vi "Measure List Report.vi"(8 "error in":errorcluster, 10 "List Number":i32(ring) items=["List 1", "List 2", "List 3", "List 4"], 11 "Instrument Handle In":i32) -> (0 "error out":errorcluster, 2 "Result":dbl[](array[numeric]), 3 "Instrument Handle Out":i32)   [LabVIEW 8.6, in "ZTScopeM.lvlib"]
doc: "Query the measurement results in a measurement list."
uses:
  ZTScopeM.lvlib
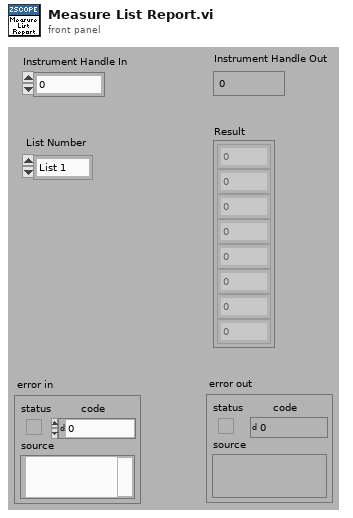
[diagram p1: front panel]
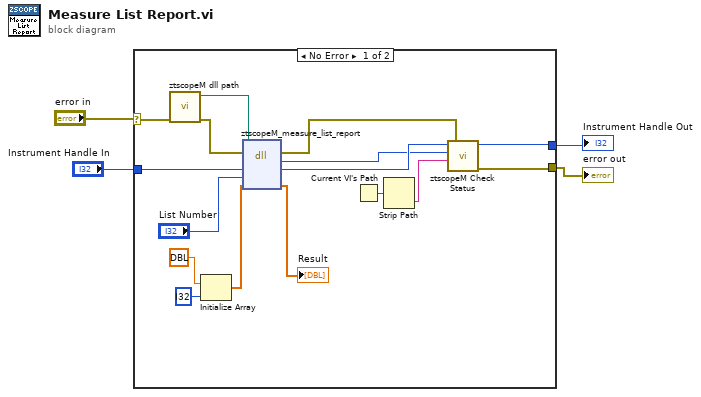
[diagram p0: block diagram]
diagram:
  n1 = case shown="No Error" "error in" {
    selector: "error in" -> [w8 w22]
    tunnel: [w13 w22] -> w1
    tunnel: [w12 w21] -> w4
    tunnel: "Instrument Handle In" -> [w19 w21]
    frame #0 {
      n2 = call "ztscopeM dll path.vi"("error in (no error)"=w8) -> ("error out"=w6:errorcluster, "<instrument>.dll path"=w7:path)  [unwired: 9 in]
      n3 = Initialize Array(dbl ?, i32 ? ("dimension size")) -> (w9:dbl[])
      n4 = dll-call lib="C:/Program Files (x86)/National Instruments/LabVIEW 2013/instr.lib/ztscopem/ztscopeM.dll" fn="ztscopeM_measure_list_report"(path in=w7, error in=w6, "instrumentHandle"=w19, "listNumber"="List Number", "result"=w9) -> (error out=w5:errorcluster, w14:i32, "instrumentHandle"=w15:i32, "result"=→"Result":dbl[])  [unwired: 2 in, 1 out]
      n5 = Current VI's Path() -> (path=w17:path)
      n6 = Strip Path(path=w17) -> (name=w16:string)  [unwired: 1 out]
      n7 = call "ztscopeM Check Status.vi"("error in"=w5, "name of VI"=w16, "status (return code)"=w14, "instrument handle in"=w15) -> ("error out"=w13:errorcluster, "instrument handle out"=w12:i32)  [unwired: 2 in]
    }
    frame #1 {
    }
  }
  "Instrument Handle Out" <- w4
  "error out" <- w1
